vi "Write states.vi"(8 "error in (no error)":errorcluster, 10 "Enum":T1, 11 "WaitPassTactic_v2 in":refnum<class "WaitPassTactic_v2.lvclass">) -> (0 "error out":errorcluster, 3 "WaitPassTactic_v2 out":refnum<class "WaitPassTactic_v2.lvclass">)   [LabVIEW 2023, in "WaitPassTactic_v2.lvclass"]
uses:
  WaitPassTactic_v2.lvclass
  WaitPassTactic_v2_states_class/WaitPassTactic_v2_states.ctl
  WaitPassTactic_v2.lvclass/WaitPassTactic_v2.ctl
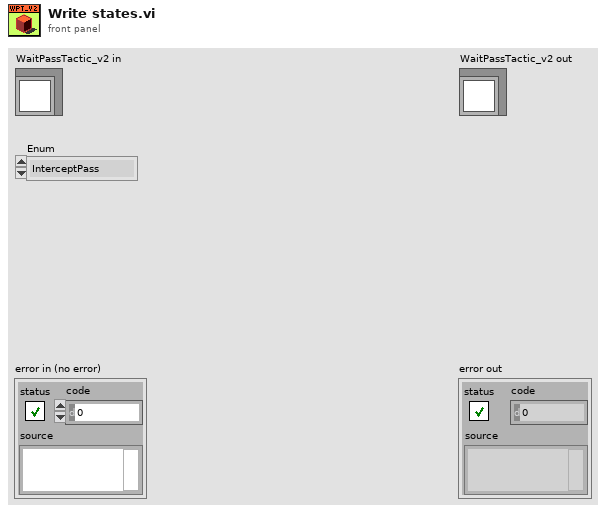
[diagram p1: front panel]
types:
  T1 = typedef "WaitPassTactic_v2.lvclass/WaitPassTactic_v2_states.ctl" = enum16{"InterceptPass\n", "OneTouchShot\n", "Exit"}
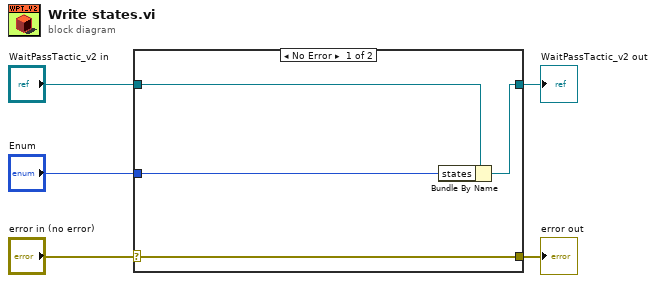
[diagram p0: block diagram]
diagram:
  n1 = case shown="No Error" "error in (no error)" {
    selector: "error in (no error)" -> [w9 w10]
    tunnel: [w9 w10] -> w4
    tunnel: [w7 w11] -> w2
    tunnel: "WaitPassTactic_v2 in" -> [w8 w11]
    tunnel: "Enum" -> [w6 _]
    frame No Error {
      n2 = Bundle By Name(cluster=w8, "states"=w6) -> (w7:refnum<class "WaitPassTactic_v2.lvclass">)
    }
    frame Error {
    }
  }
  "error out" <- w4
  "WaitPassTactic_v2 out" <- w2
